vi "Populate Cluster.vi"(7 "Prefix Name":string, 8 "error in (no error)":errorcluster, 9 "Values":string[](array[string]), 10 "Keys":string[](array[string]), 11 "Clust Refnum":refnum<vi>) -> (0 "error out":errorcluster, 3 "Cluster Refnum (Dup)":refnum<vi>)   [LabVIEW 2019]
doc: "Wire any cluster control reference to this VI, and a set of keys and values. The VI will search the key array for keys that match controls in the cluster. When it finds a match, it will populate the control with the corresponding value.\n\nSupported data types, as of 12/20/06:\nBoolean (TRUE if value is <> 0 or <> \"FALSE\")\nPath\nDouble\nString\nEnumerated Type (value can be an integer or enum string)\nTime stamp (value saved as a double)\nArray (recursive)\nCluster (recursive)\nShared Variable Reference\nRing Control (value can be an integer or ring string)\nVISA resource name\nCombo Box (value can be the string or combo box value)\n\nKey format:\n<prefix>.<control name_1>[.M.<control name_2>]...[.<control name_N>]\n\nIf the <prefix> input is an empty string, the label of the input cluster will be used instead.\n\n<control name> is the name of a control in the cluster. The control may be any supported type, including arrays and clusters.\n\n<control name_N>.n.<control name_N+1> is the Mth element of the <control name_N> array, where the array element is named <control name_N+1>. The array element name is not optional."
panel:
  in  "VI Refnum":refnum<vi>
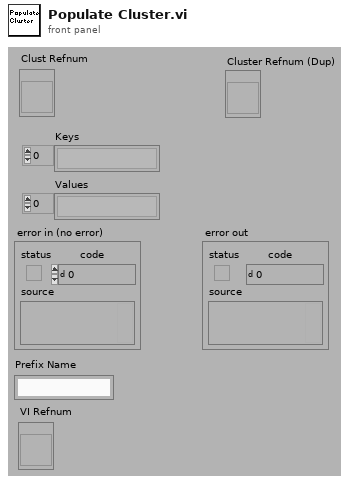
[diagram p1: front panel]
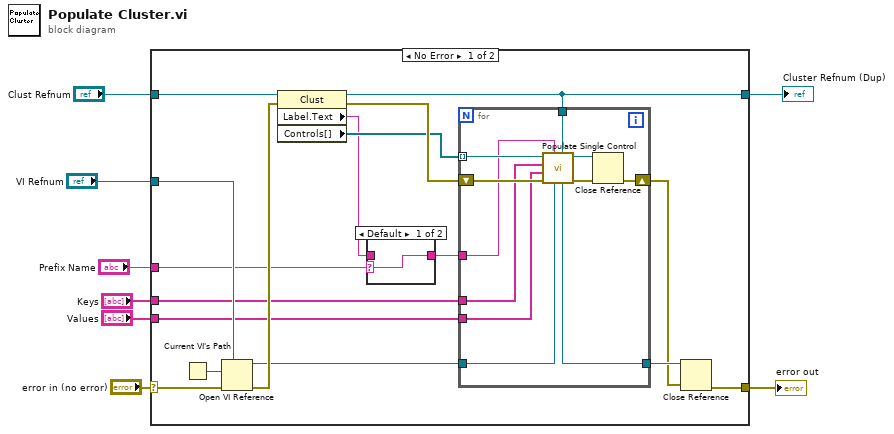
[diagram p0: block diagram]
diagram:
  n1 = case shown="No Error" "error in (no error)" {
    selector: "error in (no error)" -> [w13 w39]
    tunnel: "Clust Refnum" -> [w23 w40]
    tunnel: [w18 w40] -> w7
    tunnel: [w14 w39] -> w6
    tunnel: "VI Refnum" -> [w12 _]
    tunnel: "Prefix Name" -> [w11 _]
    tunnel: "Keys" -> [w10 _]
    tunnel: "Values" -> [w9 _]
    frame No Error {
      n2 = Current VI's Path() -> (path=w15:path)
      n3 = Open VI Reference(type specifier VI Refnum (for type only)=w12, vi path=w15, error in (no error)=w13) -> (vi reference=w19:refnum<vi>, error out=w20:errorcluster)  [unwired: 3 in]
      n4 = property class="Clust"(reference=w23, error in=w20) -> (reference out=w18:refnum<vi>, error out=w25:errorcluster, "Label.Text"=w22:string, "Controls[]"=w24:refnum<vi>[])
      n5 = case shown="Default" w11 {
        selector: w11 -> [w26 _]
        tunnel: w22 -> [_ w27]
        tunnel: [w26 w27] -> w21
        frame Default {
        }
        frame "" {
        }
      }
      n6 = for {
        tunnel: w24 -> [w38] mode=indexing
        tunnel: w10 -> [w33]
        tunnel: w9 -> [w34]
        shift-right: [w28] -> w16
        shift-left: w25 -> [w37]
        tunnel: w21 -> [w36]
        tunnel: w19 -> [w35]
        tunnel: w18 -> [w31]
        tunnel: [w32] -> w17
        n7 = call "Populate Single Control.vi"("Clust Refnum"=w31, "VI Refnum"=w35, "Prefix"=w36, "error in (no error)"=w37, "Values"=w34, "Keys"=w33, "Ctl Refnum"=w38) -> ("error out"=w30:errorcluster, "Ctl Refnum out"=w29:refnum<vi>, "VI Refnum out"=w32:refnum<vi>)  [unwired: 1 in, 1 out]
        n8 = Close Reference(reference=w29, error in (no error)=w30) -> (error out=w28:errorcluster)
      }
      n9 = Close Reference(reference=w17, error in (no error)=w16) -> (error out=w14:errorcluster)
    }
    frame Error {
    }
  }
  "error out" <- w6
  "Cluster Refnum (Dup)" <- w7
